vi "Rename Window Title to VI Name.vi"(8 "error in (no error)":errorcluster, 11 "VI Ref":refnum<vi>) -> (0 "error out":errorcluster, 2 "Save?":bool, 3 "VI Ref out":refnum<vi>)   [LabVIEW 2020, in "Code Cleanup.lvlib"]
uses:
  Code Cleanup.lvlib
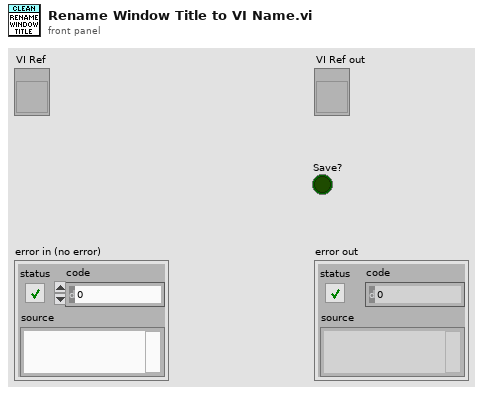
[diagram p1: front panel]
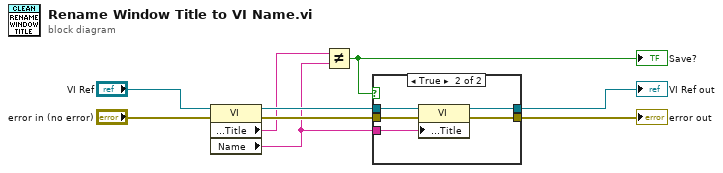
[diagram p0: block diagram]
diagram:
  n1 = property class="VI"(reference="VI Ref", error in="error in (no error)") -> (reference out=w9:refnum<vi>, error out=w8:errorcluster, "Front Panel.Title"=w7:string, "Name"=w1:string)
  n2 = Not Equal?(x=w7, y=w1) -> (x != y?=w2:bool)
  "Save?" <- w2
  n3 = case shown="True" w2 {
    tunnel: w9 -> [w10 w16]
    tunnel: w8 -> [w11 w15]
    tunnel: [w11 w14] -> w4
    tunnel: [w10 w13] -> w3
    tunnel: w1 -> [_ w12]
    frame False {
    }
    frame True {
      n4 = property class="VI"(reference=w16, error in=w15, "Front Panel.Title"=w12) -> (reference out=w13:refnum<vi>, error out=w14:errorcluster)
    }
  }
  "error out" <- w4
  "VI Ref out" <- w3
